vi "Combo.vi"(7 "Function":enum16{"Add", "Subtract", "Multiply", "Divide"}(ring), 8 "Y":dbl, 11 "X":dbl) -> (3 "Z":dbl)   [LabVIEW 2019, in "Simple Math Toolkit.lvlib"]
uses:
  Simple Math Toolkit.lvlib
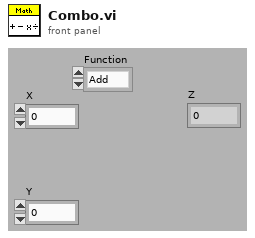
[diagram p1: front panel]
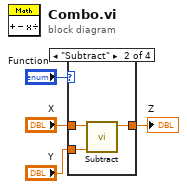
[diagram p0: block diagram]
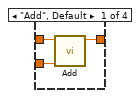
[diagram p2: hidden frame]
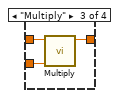
[diagram p3: hidden frame]
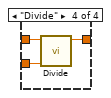
[diagram p4: hidden frame]
diagram:
  n1 = case shown="\"Subtract\"" "Function" {
    tunnel: "X" -> [w7 w9 w13 w16]
    tunnel: "Y" -> [w6 w10 w12 w15]
    tunnel: [w5 w8 w11 w14] -> w1
    frame "Add", Default {
      n2 = call "Add.vi"("Y"=w6, "X"=w7) -> ("X+Y"=w5:dbl)  [unwired: 9 in]
    }
    frame "Subtract" {
      n3 = call "Subtract.vi"("Y"=w10, "X"=w9) -> ("X-Y"=w8:dbl)  [unwired: 9 in]
    }
    frame "Multiply" {
      n4 = call "Multiply.vi"("Y"=w12, "X"=w13) -> ("X*Y"=w11:dbl)  [unwired: 9 in]
    }
    frame "Divide" {
      n5 = call "Divide.vi"("Y"=w15, "X"=w16) -> ("X/Y"=w14:dbl)  [unwired: 9 in]
    }
  }
  "Z" <- w1
